vi "Get Property.vi"(10 "Ctl Ref":refnum<vi>, 11 "Template UIP In":refnum<class "PositionUIP.lvclass">) -> (0 "Error Out":errorcluster, 3 "Template UIP Out":refnum<class "PositionUIP.lvclass">)   [LabVIEW 2015, in "PositionUIP.lvclass"]
doc: "Modify this method to implement functionality for extracting the property from VI Server Control to be stored inside UIP."
uses:
  PositionUIP.lvclass
  PositionUIP.lvclass/PositionUIP.ctl
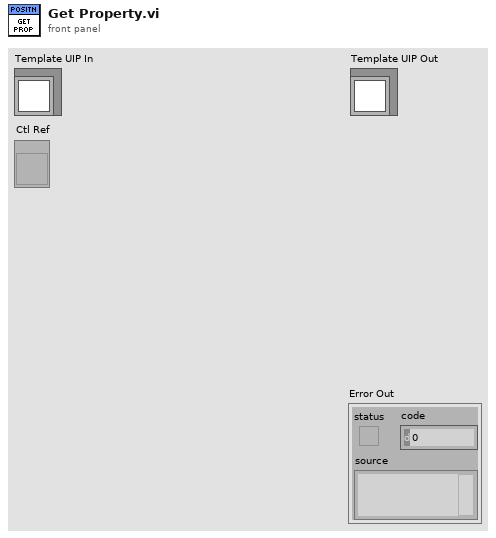
[diagram p1: front panel]
types:
  T1 = typedef "LVPositionTypeDef.ctl" = cluster{"Left":i32, "Top":i32}
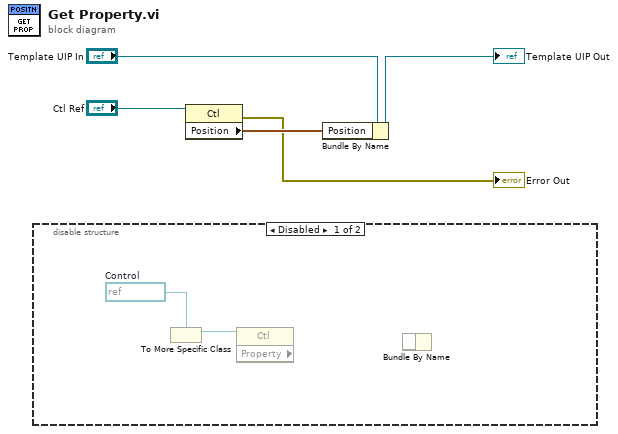
[diagram p0: block diagram]
diagram:
  n1 = disable-structure shown="Disabled" {
    frame Disabled {
      w7 = refnum<vi> refnum  # Control
      n2 = To More Specific Class(target class=w7) -> (specific class reference=w6:refnum<vi>)  [unwired: 2 in, 1 out]
      n3 = property class="Ctl" props=[](reference=w6) -> ()  [unwired: 1 in, 3 out]
      n4 = Bundle By Name "Bundle By Name"() -> ()  [unwired: 2 in, 1 out]
    }
    frame Enabled {
    }
  }
  n5 = property class="Ctl"(reference="Ctl Ref") -> (error out=→"Error Out":errorcluster, "Position"=w2:T1)  [unwired: 1 in, 1 out]
  n6 = Bundle By Name(cluster="Template UIP In", "Position"=w2) -> (→"Template UIP Out":refnum<class "PositionUIP.lvclass">)
